vi "SVFA Zoom Power Spectrum (1 Ch).vi"(0 "scaled signal [EU]":waveform(dbl)={"t0"=timestamp(0 s since 1904-01-01), "dt"=0.0001, "Y"=[]}, 3 "zoom settings":T2={"frequency range"={"start frequency"=1000.0, "stop frequency"=2000.0}, "window"=1, "number of lines"=400, "% overlap"=0.0} {"% overlap" min=0.0 format="%.2f"; "number of lines" min=2; "window" items=["None ", "Hanning", "Hamming", "Blackman-Harris", "Exact Blackman", "Blackman", "Flat Top", "4 Term B-Harris ", "7 Term B-Harris", "Low Sidelobe"]; "frequency range"."stop frequency" min=0.0 format="%.2f"; "frequency range"."start frequency" min=0.0 format="%.2f"}, 4 "dB On (T)":bool=TRUE, 5 "error in (no error)":errorcluster, 7 "averaging parameters":T1={"averaging mode"=enum."No averaging", "weighting mode"=enum."Exponential", "number of averages"=10, "linear mode"=enum."One shot"} {"number of averages" min=1 step=1}, 9 "restart averaging (F)":bool) -> (11 "averaging done":bool, 12 "new spectrum available":bool, 13 "averages completed":dbl, 14 "power spectrum [dB EU]":cluster{"f0":dbl, "df":dbl, "magnitude":dbl[]}={"f0"=nan, "df"=inf, "magnitude"=[]} {"magnitude" format="%.2p"; "df" format="%.2p"; "f0" format="%.2p"}, 15 "unit label":string, 18 "spectrum info":T3={"channel name"="", "description"="", "x-axis units"=1, "spectral info"={"spectrum type"=enum."Power [Magnitude^2]", "linear/dB"=enum."linear", "window"=0, "window size"=0, "FFT size"=0}, "engineering units"=0, "custom label"="", "dB reference [EU]"=0.0, "peak units"=enum."rms", "weighting filter"=0, "spectral density?"=FALSE, "unit label"="", "spectrum skewed?"=FALSE, "complimentary spectrum units"=enum."none"} {"x-axis units" items=["Time (s)"=0, "Frequency-CB (Hz)"=1, "Frequency-CPB (Hz)"=1248, "Frequency-Arbitrary (Hz)"=2357, "Quefrency (s)"=2, "Revolutions (rev)"=3, "Order"=4, "Speed (RPM)"=11, "Speed (rad/s)"=21, "Index"=65535]; "weighting filter" items=["Linear", "A-weighting", "B-weighting", "C-weighting", "ITU-R 468-4", "Dolby", "CCITT", "C-message", "Wb", "Wc", "Wd", "We", "Wf", "Wh", "Wj", "Wk", "Wm", "AES17 20 kHz lowpass", "AES17 40 kHz lowpass", "AES17 20 kHz highpass", "AES17 40 kHz highpass"]; "dB reference [EU]" format="%.2f"; "engineering units" items=["custom..."=0, "V"=1, "A"=21, "C"=30, "pC"=31, "s"=32, "-"=29, "Pa"=2, "N"=20, "g"=3, "m/s^2"=4, "m/s"=5, "m"=6, "mm/s"=12, "mm"=13, "micron/s"=14, "micron"=15, "in/s^2"=7, "in/s"=8, "in"=9, "mil/s"=10, "mil"=11, "rad/s^2"=16, "rad/s"=17, "rad"=18, "deg/s^2"=26, "deg/s"=27, "deg"=28, "RPM"=22, "cycle/s^2"=23, "Hz"=24, "cycle"=25, "strain"=19]; "spectral info"."window" items=["None "=0, "Hanning"=1, "Hamming"=2, "Blackman-Harris"=3, "Exact Blackman"=4, "Blackman"=5, "Flat Top"=6, "4 Term B-Harris "=7, "7 Term B-Harris"=8, "Low Sidelobe"=9, "Force - Exponential"=10, "Gaussian"=62]}, 19 "error out":errorcluster)   [LabVIEW 2017]
doc: "Computes the zoom power spectrum of <B>scaled signal [EU]</B> and <B>zoom settings</B>. Data accumulates each time this VI is called. However, it returns a new spectrum only when sufficient data accumulates. Indicators and subsequent processing should only be called when <B>new spectrum available</B> is TRUE. Wire data to the <B>scaled signal [EU]</B> input to determine the polymorphic instance to use or manually select the instance."
uses:
  <vilib>/addons/_NISVFA/_Shared subVIs/Controls/svc_Spectrum Info.ctl
  <vilib>/addons/_NISVFA/_Shared subVIs/Controls/svc_X-Axis Units.ctl
  <vilib>/addons/_NISVFA/_Shared subVIs/Controls/svc_Spectrum Type.ctl
  <vilib>/addons/_NISVFA/_Shared subVIs/Controls/svc_Engineering Units Text Ring.ctl
  <vilib>/addons/_NISVFA/_Shared subVIs/Controls/svc_Weighting Filter Text Ring.ctl
  <vilib>/addons/_NISVFA/_Shared subVIs/Controls/svc_Complimentary Spectrum Units.ctl
  <vilib>/addons/_NISVFA/_Shared subVIs/Common/svc_Get SV Channel Info.vi
  <vilib>/addons/_NISVFA/_Shared subVIs/Common/svc_Spectrum Units.vi
  <vilib>/addons/_NISVFA/_Shared subVIs/Spectrum Averaging/svfa_Reset Averaging State Info.vi
  <vilib>/addons/_NISVFA/_Shared subVIs/Spectrum Averaging/svfa_Average Array with Avg Checks (complex) No State.vi
  <vilib>/addons/_NISVFA/_Shared subVIs/Common/svc_Complex to Mag2 Array.vi
  <vilib>/addons/_NISVFA/_Shared subVIs/Spectrum Averaging/svfa_Average Array with Avg Checks (real) No State.vi
  <vilib>/addons/_NISVFA/_Shared subVIs/Spectrum Averaging/svfa_Average Array (complex) No State.vi
  <vilib>/addons/_NISVFA/_Shared subVIs/Spectrum Averaging/svfa_Average Array (real) No State.vi
  <vilib>/addons/_NISVFA/_Shared subVIs/Spectrum Averaging/svfa_No Average Array (complex).vi
  <vilib>/addons/_NISVFA/_Shared subVIs/Spectrum Averaging/svfa_Average Array (complex).vi
  <vilib>/addons/_NISVFA/_Shared subVIs/Spectrum Averaging/svfa_No Average Array (real).vi
  <vilib>/addons/_NISVFA/_Shared subVIs/Spectrum Averaging/svfa_Average Array (real).vi
  <vilib>/addons/_NISVFA/_Shared subVIs/Spectrum Averaging/svfa_Peak Hold Array.vi
  <vilib>/addons/_NISVFA/_Shared subVIs/Common/svc_Get Weighting Enum and Labels.vi
  <vilib>/addons/_NISVFA/_Shared subVIs/Common/svc_Unit Label Lexical Class.vi
  <vilib>/addons/_NISVFA/_Shared subVIs/Common/svc_Engineering Units to Unit Label.vi
  <vilib>/addons/_NISVFA/_Shared subVIs/Common/svc_Format Value (DBL).vi
  <vilib>/addons/_NISVFA/_Shared subVIs/Common/svc_Channel Info to Spectrum Info.vi
  <vilib>/addons/_NISVFA/_Shared subVIs/Common/svc_Unit Label to Engineering Units.vi
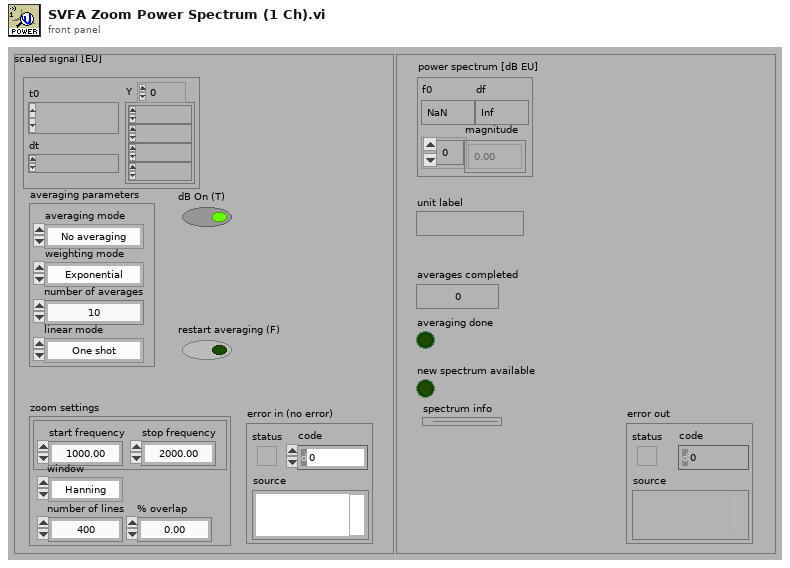
[diagram p1: front panel]
types:
  T1 = cluster{"averaging mode":enum16{"No averaging", "Vector averaging", "RMS averaging", "Peak hold"}, "weighting mode":enum16{"Linear", "Exponential"}, "number of averages":u32, "linear mode":enum16{"One shot", "Auto restart"}}
  T2 = cluster{"frequency range":cluster{"start frequency":dbl, "stop frequency":dbl}, "window":u16, "number of lines":i32, "% overlap":dbl}
  T3 = typedef "svc_Spectrum Info.ctl" = cluster{"channel name":string, "description":string, "x-axis units":T4, "spectral info":cluster{"spectrum type":T5, "linear/dB":enum16{"linear", "dB"}, "window":u16, "window size":i32, "FFT size":i32}, "engineering units":T6, "custom label":string, "dB reference [EU]":dbl, "peak units":enum16{"rms", "peak", "peak-peak"}, "weighting filter":T7, "spectral density?":bool, "unit label":string, "spectrum skewed?":bool, "complimentary spectrum units":T8}
  T4 = typedef "svc_X-Axis Units.ctl" = u16
  T5 = typedef "svc_Spectrum Type.ctl" = enum16{"FFT Spectrum [complex]", "Amplitude [Magnitude]", "Power [Magnitude^2]", "Cross Spectrum [complex]", "Frequency Response [Complex]"}
  T6 = typedef "svc_Engineering Units Text Ring.ctl" = u16
  T7 = typedef "svc_Weighting Filter Text Ring.ctl" = u16
  T8 = typedef "svc_Complimentary Spectrum Units.ctl" = enum16{"none", "radians", "degrees", "cycles", "imaginary"}
  T9 = enum16{"Restart processing", "Continue processing", "Skip processing"}
  T10 = enum16{"No averaging", "Vector averaging", "RMS averaging", "Peak hold"}
  T11 = cluster{"complex FFT":cdb[], "real FFT":dbl[], "f0":dbl, "df":dbl, "averages completed":dbl, "averaging parameters":cluster{"averaging mode":enum16{"No averaging", "Vector averaging", "RMS averaging", "Peak hold"}, "weighting mode":enum16{"Linear", "Exponential"}, "number of averages":u32, "linear mode":enum16{"One shot", "Auto restart"}}}
  T12 = cluster{"zoom settings":cluster{"center frequency":dbl, "zoom":i32, "trim":dbl}, "FFT settings":cluster{"window":enum16{"None ", "Hanning", "Hamming", "Blackman-Harris", "Exact Blackman", "Blackman", "Flat Top", "4 Term B-Harris ", "7 Term B-Harris", "Low Sidelobe"}, "window size":i32, "FFT size":i32, "%overlap":dbl}}
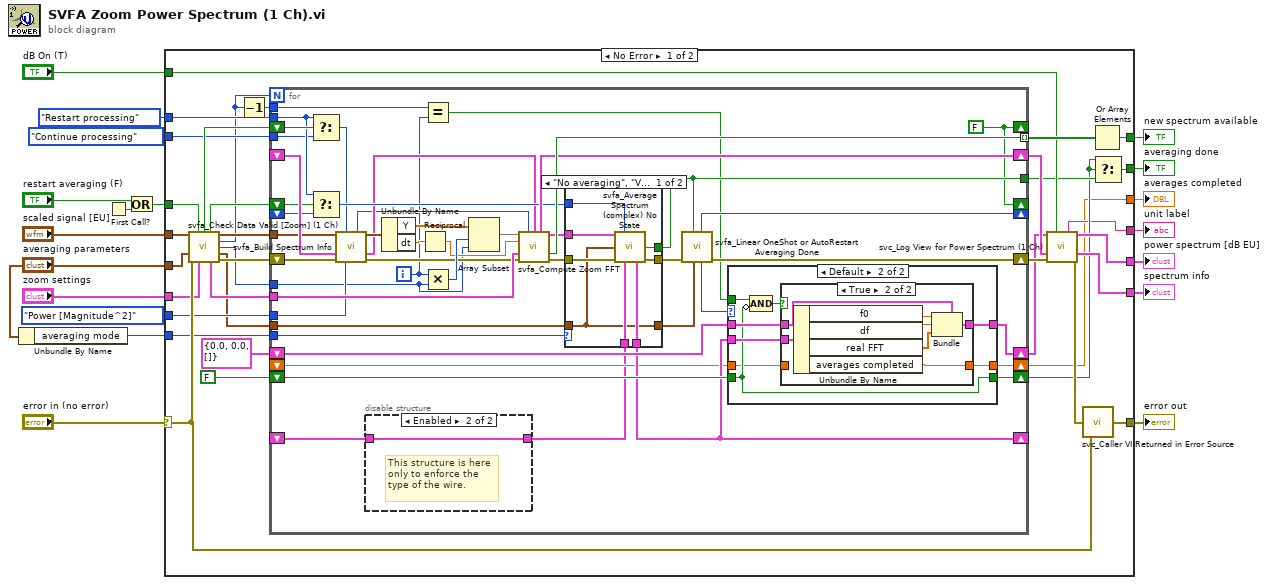
[diagram p0: block diagram]
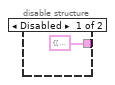
[diagram p2: hidden frame]
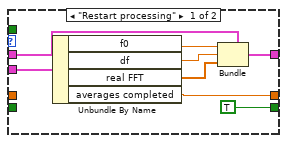
[diagram p3: hidden frame]
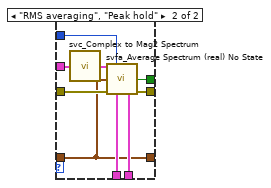
[diagram p5: hidden frame]
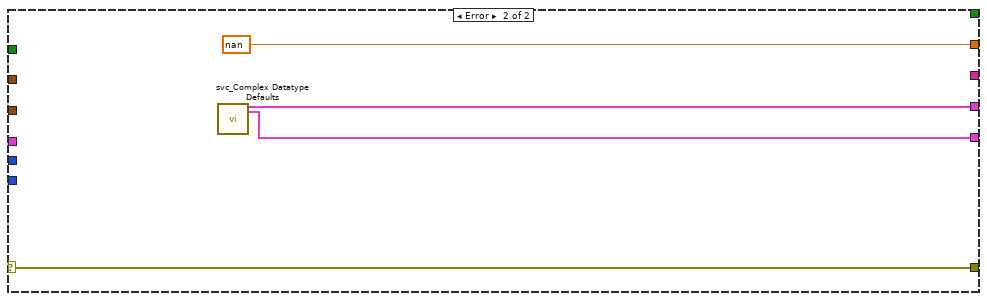
[diagram p6: hidden frame]
diagram:
  n1 = Unbundle By Name("averaging parameters") -> ("averaging mode"=w1:T10)
  n2 = First Call?() -> (First Call?: T/F=w8:bool)
  n3 = Or(x="restart averaging (F)", y=w8) -> (x .or. y?=w6:bool)
  n4 = case shown="No Error" "error in (no error)" {
    selector: "error in (no error)" -> [w48 w148]
    tunnel: w6 -> [w38 _]
    tunnel: [w21 nan ("Averaged So-far")] -> w19
    tunnel: [w39 _] -> w18
    tunnel: [w53 w146] -> w14
    tunnel: [w49 w148] -> w17
    tunnel: "averaging parameters" -> [w50 _]
    tunnel: "zoom settings" -> [w45 _]
    tunnel: "scaled signal [EU]" -> [w54 _]
    tunnel: [w22 _] -> w13
    tunnel: "dB On (T)" -> [w41 _]
    tunnel: [w51 w145] -> w12
    tunnel: [w29 _] -> w10
    tunnel: T9."Restart processing" ("processing control") -> [w35 _]
    tunnel: T9."Continue processing" ("processing control") -> [w34 _]
    tunnel: svc_Spectrum_Type."Power [Magnitude^2]" ("spectrum type") -> [w33 _]
    tunnel: w1 -> [w20 _]
    frame No Error {
      n5 = call <vilib>:"svfa_Check Data Valid [Zoom] (1 Ch).vi"("signal [V]"=w54, "restart averaging (F)"=w38, "averaging parameters"=w50, "error in (no error)"=w48, "zoom settings"=w45) -> ("reset processing"=w36:bool, "restart averaging"=w37:bool, "dup signal [V]"=w47:waveform(dbl), "iterations"=w31:i32, "maximum block size"=w40:i32, "dup averaging parameters"=w24:T1, "zoom FFT settings"=w44:T12, "error out"=w46:errorcluster)  [unwired: 3 in]
      n6 = Decrement(x=w31) -> (x-1=w30:i32)
      n7 = for {
        N: w31 -> [_]
        tunnel: [w99] -> w43 mode=indexing
        tunnel: w47 -> [w90]
        tunnel: [w100] -> w26
        shift-left: _ -> [w56]
        shift-right: [w60] -> _
        shift-right: [w97] -> w42
        shift-left: _ -> [w96]
        tunnel: w24 -> [w71]
        shift-right: [w69] -> _
        shift-left: _ -> [w95]
        tunnel: w44 -> [w92]
        shift-right: [w85] -> _
        shift-left: w37 -> [w94]
        tunnel: w40 -> [w66]
        shift-right: [w98] -> w32
        shift-left: w46 -> [w89]
        shift-right: [w85] -> _
        shift-left: w36 -> [w88]
        tunnel: w35 -> [w87]
        tunnel: w34 -> [w86]
        tunnel: w33 -> [w72]
        shift-right: [w68] -> w25
        shift-left: FALSE ("restart averaging") -> [w65]
        shift-right: [w67] -> w23
        shift-left: cluster{"f0":dbl, "df":dbl, "real FFT":dbl[]} {"f0"=0.0, "df"=0.0, "real FFT"=[]} -> [w61]
        tunnel: w30 -> [w63]
        tunnel: w20 -> [w59]
        shift-right: [w58] -> w21
        shift-left: _ -> [w57]
        i -> [w64]
        w85 = FALSE ("restart averaging")
        n8 = Select(t=w87, s=w88, f=w86) -> (s? t:f=w84:T9)
        n9 = Select(t=w87, s=w94, f=w95) -> (s? t:f=w93:T9)
        n10 = call <vilib>:"svfa_Build Spectrum Info.vi"("scaled signal [EU]"=w90, "processing control"=w84, "spectrum info in"=w96, "error in (no error)"=w89, "spectrum type"=w72) -> ("dup processing control"=w73:T9, "dup scaled signal [EU]"=w82:waveform(dbl), "spectrum info out"=w80:T3, "error out"=w76:errorcluster)  [unwired: 7 in]
        n11 = disable-structure shown="Enabled" {
          disable-tunnel: w56 -> [_ w102]
          disable-tunnel: [T11 {"complex FFT"=[], "real FFT"=[], "f0"=0.0, "df"=0.0, "averages completed"=0.0, "averaging parameters"={"averaging mode"=enum."No averaging", "weighting mode"=enum."Linear", "number of averages"=10, "linear mode"=enum."Auto restart"}} ("averaging state info in") w102] -> w55
          frame Disabled {
          }
          frame Enabled {
            # "This structure is here\nonly to enforce the\ntype of the wire."
          }
        }
        n12 = Unbundle By Name ("Get Waveform Components")(w82) -> ("Y"=w79:dbl[], "dt"=w81:dbl)
        n13 = Reciprocal(x=w81) -> (1/x=w74:dbl)
        n14 = Equal?(x=w63, y=w64) -> (x = y?=w62:bool)
        n15 = Multiply(x=w64, y=w66) -> (x*y=w91:i32)
        n16 = Array Subset(array=w79, index=w91, length=w66) -> (w75:dbl[])
        n17 = call <vilib>:"svfa_Compute Zoom FFT.vi"("x"=w75, "processing control"=w73, "spectrum info"=w80, "fs"=w74, "zoom FFT settings"=w92, "error in (no error)"=w76) -> ("spectrum info out"=w97:T3, "FFT spectrum"=w78:cluster{"f0":dbl, "df":dbl, "spectrum":cdb[]}, "spectrum ready"=w99:bool, "error out"=w77:errorcluster)  [unwired: 5 in, 1 out]
        n18 = case shown="\"No averaging\", \"Vector averaging\"" w59 {
          tunnel: w71 -> [w128 w136]
          tunnel: [w133 w142] -> w83
          tunnel: [w132 w143] -> w100
          tunnel: w78 -> [w135 w141]
          tunnel: w77 -> [w134 w144]
          tunnel: w93 -> [w131 w139]
          tunnel: w55 -> [w130 w137]
          tunnel: [w129 w138] -> w60
          tunnel: [w128 w136] -> w70
          frame "No averaging", "Vector averaging" {
            n19 = call <vilib>:"svfa_Average Spectrum (complex) No State.vi"("spectrum"=w135, "processing control"=w131, "averaging parameters"=w128, "error in (no error)"=w134, "averaging state info in"=w130) -> ("averaging done"=w132:bool, "averaging state info out"=w129:T11, "error out"=w133:errorcluster)  [unwired: 5 in, 3 out]
          }
          frame "RMS averaging", "Peak hold" {
            n20 = call <vilib>:"svc_Complex to Mag2 Spectrum.vi"("complex spectrum"=w141) -> ("power spectrum"=w140:cluster{"f0":dbl, "df":dbl, "spectrum":dbl[]})  [unwired: 4 in]
            n21 = call <vilib>:"svfa_Average Spectrum (real) No State.vi"("spectrum"=w140, "processing control"=w139, "averaging parameters"=w136, "error in (no error)"=w144, "averaging state info in"=w137) -> ("averaging done"=w143:bool, "averaging state info out"=w138:T11, "error out"=w142:errorcluster)  [unwired: 5 in, 3 out]
          }
        }
        n22 = call <vilib>:"svfa_Linear OneShot or AutoRestart Averaging Done.vi"("averaging parameters"=w70, "averaging done"=w100, "error in (no error)"=w83) -> ("error out"=w98:errorcluster, "processing control"=w69:T9)  [unwired: 7 in]
        n23 = case shown="Default" w69 {
          tunnel: w60 -> [w107 w118]
          tunnel: [TRUE ("restart averaging") w113] -> w68
          tunnel: [w105 w117] -> w67
          tunnel: w65 -> [_ w113]
          tunnel: w62 -> [_ w116]
          tunnel: w61 -> [w104 w115]
          tunnel: [w103 w112] -> w58
          tunnel: w57 -> [_ w111]
          frame "Restart processing" {
            n24 = Unbundle By Name(w107) -> ("f0"=w110:dbl, "df"=w109:dbl, "real FFT"=w108:dbl[], "averages completed"=w103:dbl)
            n25 = Bundle(cluster=w104, "f0"=w110, "df"=w109, "real FFT"=w108) -> (w105:cluster{"f0":dbl, "df":dbl, "real FFT":dbl[]})
          }
          frame Default {
            n26 = Compound Arithmetic op=AND(w116, invert w113) -> (w114:bool)
            n27 = case shown="True" w114 {
              tunnel: w118 -> [_ w124]
              tunnel: [w120 w123] -> w117
              tunnel: w115 -> [w120 w122]
              tunnel: [w119 w121] -> w112
              tunnel: w111 -> [w119 _]
              frame False {
              }
              frame True {
                n28 = Unbundle By Name(w124) -> ("f0"=w127:dbl, "df"=w126:dbl, "real FFT"=w125:dbl[], "averages completed"=w121:dbl)
                n29 = Bundle(cluster=w122, "f0"=w127, "df"=w126, "real FFT"=w125) -> (w123:cluster{"f0":dbl, "df":dbl, "real FFT":dbl[]})
              }
            }
          }
        }
      }
      n30 = call <vilib>:"svc_Log View for Power Spectrum (1 Ch).vi"("power spectrum [dB EU]"=w23, "dB On (T)"=w41, "spectrum info"=w42, "error in (no error)"=w32) -> ("unit label"=w22:string, "power spectrum [dB EU]"=w53:cluster{"f0":dbl, "df":dbl, "magnitude":dbl[]}, "spectrum info out"=w51:T3, "error out"=w52:errorcluster)  [unwired: 8 in]
      n31 = call <vilib>:"svc_Caller VI Returned in Error Source.vi"("warning input to caller"=w48, "error in (no error)"=w52) -> ("error out"=w49:errorcluster)  [unwired: 3 in]
      n32 = Or Array Elements(Boolean array=w43) -> (logical OR=w39:bool)
      n33 = Select(t=w25, s=w25, f=w26) -> (s? t:f=w29:bool)
    }
    frame Error {
      n34 = call <vilib>:"svc_Complex Datatype Defaults.vi"() -> ("empty spectrum"=w146:cluster{"f0":dbl, "df":dbl, "magnitude":dbl[]}, "dead spectrum info"=w145:T3)  [unwired: 11 in, 7 out]
    }
  }
  "averages completed" <- w19
  "new spectrum available" <- w18
  "error out" <- w17
  "power spectrum [dB EU]" <- w14
  "unit label" <- w13
  "spectrum info" <- w12
  "averaging done" <- w10
